vi "Send API Request v4.vi"(5 "AWS Core":refnum<class "NI_AWS_Core.lvclass">, 6 "request body":string, 7 "Authorization":string, 8 "error in (no error)":errorcluster, 9 "HTTP-Verb":string, 10 "Host String":string, 11 "Client Handle":T1) -> (0 "error out":errorcluster, 1 "Call Result":string, 2 "response body":string, 3 "response headers":string, 4 "Redirect endpoint":string)   [LabVIEW 2015, in "NI_AWS_Core.lvclass"]
uses:
  NI_AWS_Core.lvclass
  <vilib>/httpClient/ClientHandle.ctl
  <vilib>/httpClient/PUTBuffer.vi
  <vilib>/httpClient/POSTBuffer.vi
  <vilib>/httpClient/LabVIEWHTTPClient.lvlib
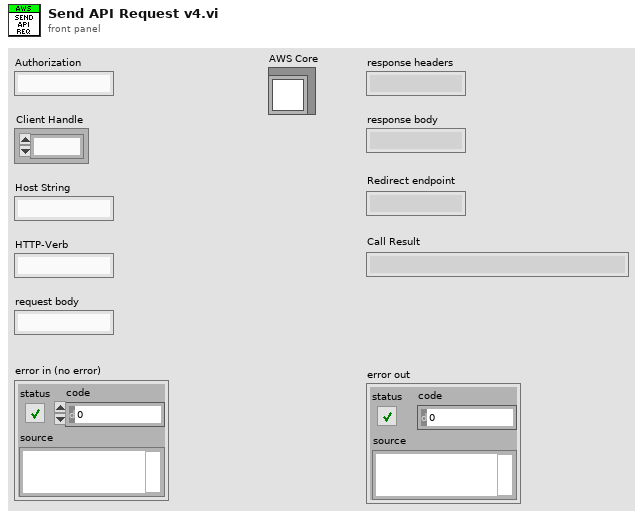
[diagram p1: front panel]
types:
  T1 = typedef "LabVIEWHTTPClient.lvlib/ClientHandle.ctl" = refnum<k1>
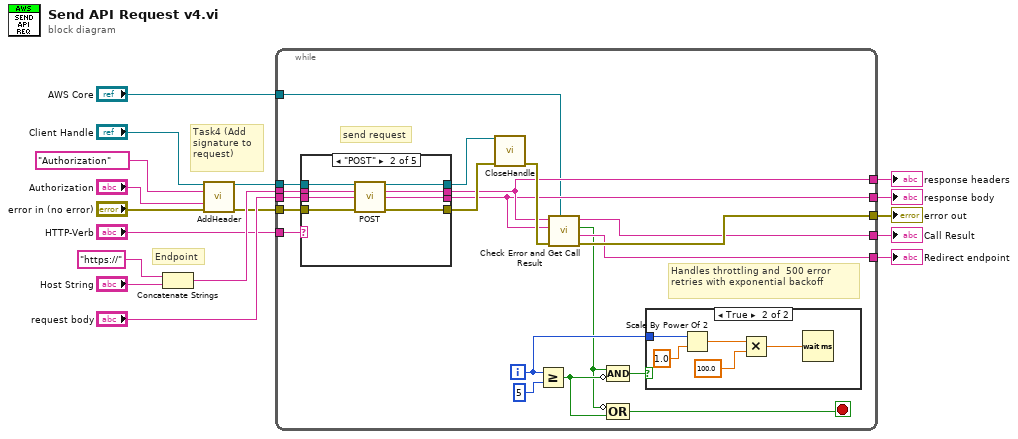
[diagram p0: block diagram]
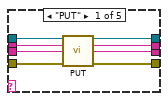
[diagram p2: hidden frame]
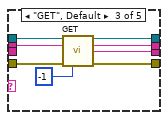
[diagram p3: hidden frame]
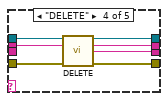
[diagram p4: hidden frame]
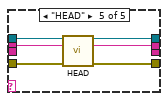
[diagram p5: hidden frame]
diagram:
  # "Endpoint"
  # "Task4 (Add signature to request)"
  n1 = Concatenate Strings("https://" ("string"), "Host String") -> (w16:string)
  n2 = call <vilib>:"AddHeader.vi"("client handle"="Client Handle", "header"="Authorization", "value"="Authorization", "error in (no error)"="error in (no error)") -> ("client handle out"=w10:T1, "error out"=w13:errorcluster)  [unwired: 10 in]
  n3 = while {
    tunnel: w10 -> [w34]
    tunnel: [w19] -> w2
    tunnel: w16 -> [w36]
    tunnel: [w24] -> w5
    tunnel: "request body" -> [w37]
    tunnel: [w23] -> w4
    tunnel: "HTTP-Verb" -> [w33]
    tunnel: [w21] -> w3
    tunnel: w13 -> [w35]
    tunnel: [w30] -> w6
    tunnel: "AWS Core" -> [w18]
    i -> [w28]
    stop <- w27 stop-if-true
    # "Handles throttling and  500 error retries with exponential backoff"
    # "send request"
    n4 = case shown="\"POST\"" w33 {
      tunnel: [w40 w53 w60 w63 _] -> w23
      tunnel: [w39 w52 w61 w62 w74] -> w24
      tunnel: w36 -> [w44 w51 w57 w66 w72]
      tunnel: w34 -> [w45 w50 w56 w65 w70]
      tunnel: w37 -> [w43 w49 _ _ _]
      tunnel: w35 -> [w42 w48 w58 w67 w71]
      tunnel: [w41 w47 w59 w68 w73] -> w31
      tunnel: [w38 w46 w55 w64 w69] -> w32
      frame "PUT" {
        n5 = call-poly <vilib>:"PUT.vi"("client handle"=w45, "url"=w44, "buffer"=w43, "error in (no error)"=w42) -> ("client handle out"=w38:T1, "headers"=w39:string, "body"=w40:string, "error out"=w41:errorcluster)  [unwired: 8 in]
      }
      frame "POST" {
        n6 = call-poly <vilib>:"POST.vi"("client handle"=w50, "url"=w51, "buffer"=w49, "error in (no error)"=w48) -> ("client handle out"=w46:T1, "headers"=w52:string, "body"=w53:string, "error out"=w47:errorcluster)  [unwired: 8 in]
      }
      frame "GET", Default {
        n7 = call <vilib>:"GET.vi"("client handle"=w56, "url"=w57, "error in (no error)"=w58, "timeout (10000)"=-1) -> ("client handle out"=w55:T1, "headers"=w61:string, "body"=w60:string, "error out"=w59:errorcluster)  [unwired: 8 in]
      }
      frame "DELETE" {
        n8 = call <vilib>:"DELETE.vi"("client handle"=w65, "url"=w66, "error in (no error)"=w67) -> ("client handle out"=w64:T1, "headers"=w62:string, "body"=w63:string, "error out"=w68:errorcluster)  [unwired: 9 in]
      }
      frame "HEAD" {
        n9 = call <vilib>:"HEAD.vi"("client handle"=w70, "url"=w72, "error in (no error)"=w71) -> ("client handle out"=w69:T1, "headers"=w74:string, "error out"=w73:errorcluster)  [unwired: 10 in]
      }
    }
    n10 = call <vilib>:"CloseHandle.vi"("client handle"=w32, "error in (no error)"=w31) -> ("error out"=w29:errorcluster)  [unwired: 13 in]
    n11 = Greater Or Equal?(x=w28, y=5) -> (x >= y?=w25:bool)
    n12 = call "Check Error and Get Call Result.vi"("AWS Core"=w18, "error in (no error)"=w29, "Response body"=w23, "Response header"=w24) -> ("error out"=w30:errorcluster, "Redirect endpoint"=w21:string, "500 Or Throttled?"=w20:bool, "Call Result"=w19:string)  [unwired: 4 in]
    n13 = Compound Arithmetic op=AND(w20, invert w25) -> (w26:bool)
    n14 = Compound Arithmetic op=OR(invert w20, w25) -> (w27:bool)
    n15 = case shown="True" w26 {
      tunnel: w28 -> [_ w78]
      frame False {
        # "Do not reattempt call"
      }
      frame True {
        n16 = Scale By Power Of 2(n=w78, x=1.0) -> (x*2^n=w76:dbl)
        n17 = Multiply(x=w76, y=100.0) -> (x*y=w77:dbl)
        n18 = Wait (ms)(milliseconds to wait=w77) -> ()  [unwired: 1 out]
      }
    }
  }
  "response headers" <- w5
  "response body" <- w4
  "error out" <- w6
  "Redirect endpoint" <- w3
  "Call Result" <- w2
